vi "FP_Size VI to Deoration Index.vi"(8 "Error":errorcluster, 9 "FPSet":T1={"Menu Bar"=FALSE, "Position"=enum."MID-CTR", "Decoration index"=0, "border(px)"=-2, "Monitor #"=0}, 11 "VI Ref":refnum<vi>) -> (0 "Error Out":errorcluster, 3 "VI Ref Out":refnum<vi>)   [LabVIEW 2020]
doc: "sets up a fp to center of monitor 1 around largest decoration. shows scroll bars if developing and hides them if not."
uses:
  TypeDefs_Utility/Cluster_FP Set.ctl
  TypeDefs_Utility/ENUM RB_Pos_Quadrant Position.ctl
  FPClass/DecFrame_FP/DecFrame_FP.lvclass
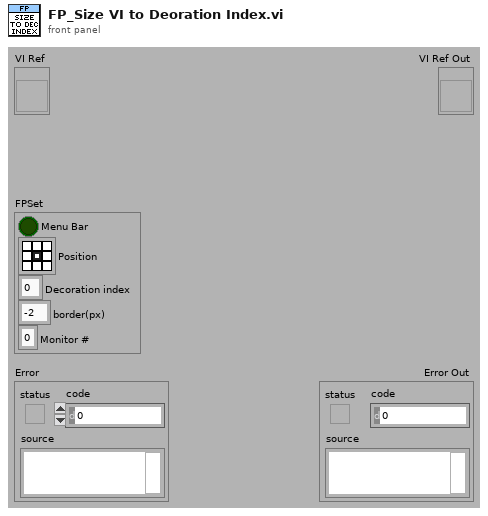
[diagram p1: front panel]
types:
  T1 = typedef "Cluster_FP Set.ctl" = cluster{"Menu Bar":bool, "Position":T2, "Decoration index":i32, "border(px)":i32, "Monitor #":i32}
  T2 = typedef "ENUM RB_Pos_Quadrant Position.ctl" = enum32{"LFT-TOP", "MID-TOP", "RGT-TOP", "LFT-CTR", "MID-CTR", "RGT-CTR", "LFT-BOT", "MID-BOT", "RGT-BOT"}
  T3 = enum32{"Invalid", "Standard", "Closed", "Hidden", "Minimized", "Maximized"}
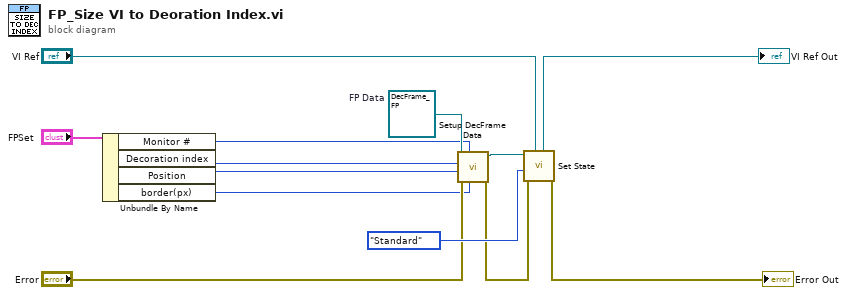
[diagram p0: block diagram]
diagram:
  w13 = refnum<class "DecFrame_FP.lvclass"> refnum  # FP Data
  n1 = Unbundle By Name("FPSet") -> ("Monitor #"=w4:i32, "Decoration index"=w3:i32, "Position"=w2:T2, "border(px)"=w1:i32)
  n2 = call-dynamic "Setup DecFrame Data.vi"("Border Spacing"=w1, "Monitor Select"=w4, "Error"="Error", "FPLocation"=w2, "Decoration Index"=w3, "FP"=w13) -> ("Error Out"=w9:errorcluster, "FP Out"=w11:refnum<class "DecFrame_FP.lvclass">)  [unwired: 4 in]
  n3 = call-dynamic "Set State.vi"("VI Ref"="VI Ref", "Error"=w9, "State"=T3."Standard", "FP"=w11) -> ("Error Out"=→"Error Out":errorcluster, "VI Ref"=→"VI Ref Out":refnum<vi>)  [unwired: 5 in, 1 out]
